vi "Wrapper_openAllSpectrometers.vi"(0 "Wrapper In":u32) -> (1 "Number of Spectrometers":i32, 2 "Wrapper Out":u32)   [LabVIEW 2017]
uses:
  OmniDriver32.dll
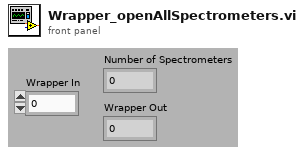
[diagram p1: front panel]
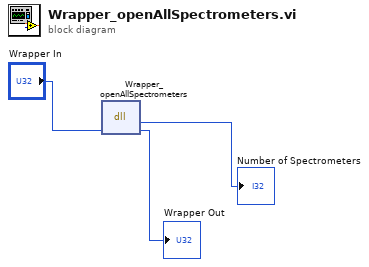
[diagram p0: block diagram]
diagram:
  n1 = dll-call lib="OmniDriver32.dll" fn="Wrapper_openAllSpectrometers" label="Wrapper.openAllSpectrometers"("Wrapper"="Wrapper In") -> (→"Number of Spectrometers":i32, "Wrapper"=→"Wrapper Out":u32)  [unwired: 3 in, 2 out]
